vi "Simple Frequency Reader.vi"(8 "error in (no error)":errorcluster) -> (0 "error out":errorcluster)   [LabVIEW 2013]
uses:
  <vilib>/Platform/TimedLoop/XDataNode/wakeup.ctl
  <vilib>/Platform/TimedLoop/XDataNode/XDNodeRunTimeDep.lvlib
  <vilib>/Platform/TimedLoop/XDataNode/nitl_modes.ctl
  <vilib>/Platform/TimedLoop/XDataNode/timing_clust.ctl
  <vilib>/platform/TimedLoop/XDataNode/XDataNode.xnode
  PMU Recorder Light/PMU Recorder Light.lvlib
panel:
  out "Waveform Chart":waveform(sgl)[](graph)
  in  "stop":bool
  in  "Refresh Rate":i64(ring)=200 items=["50 Hz"=20, "20 Hz"=50, "10 Hz"=100, "5 Hz"=200, "2 Hz"=500, "1 Hz"=1000, "Every 2 sec"=2000, "Every 5 sec"=5000, "Every 10 sec"=10000, "Every minute"=60000]
  # "INPUT"
  # "INTERMEDIATE"
  # "OUTPUT"
  # "USAGE:  Start the PRL, configure the input PDC address (IP/Port/PDC ID), press startup and wait until it is connected. \nThen start this VI."
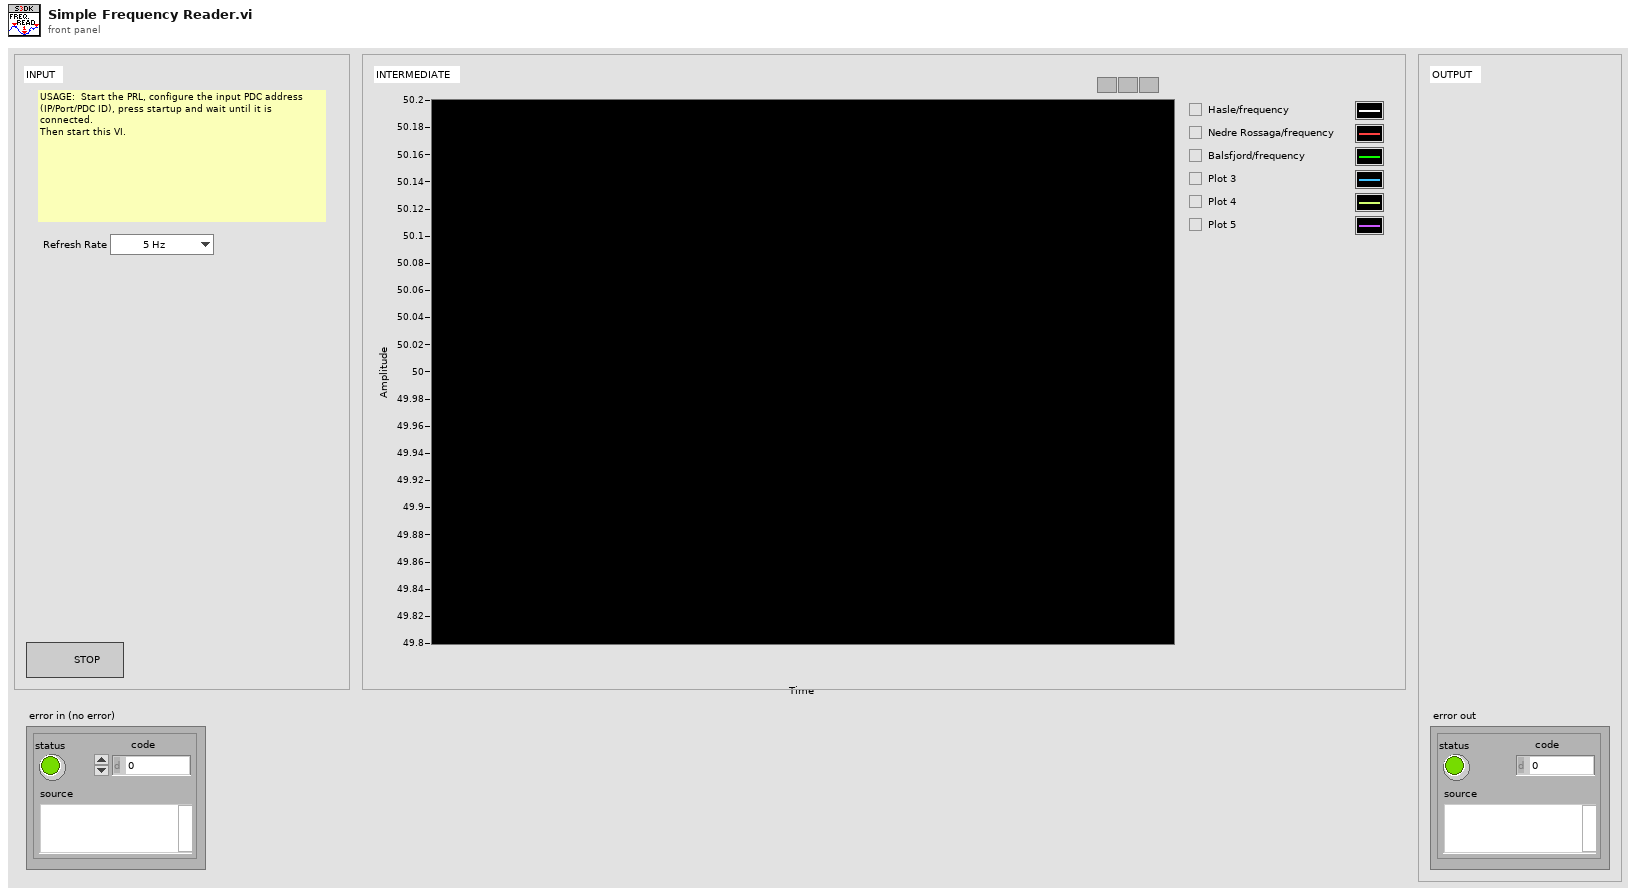
[diagram p1: front panel]
types:
  T1 = enum16{"Filter Signals", "Get All Signal Names", "Select Signals on Name", "Select Frequency Only", "Get Selected Signal Names"}
  T2 = typedef "XDNodeRunTimeDep.lvlib/timing_clust.ctl" = cluster{"Expected End [f-1]":u64, "Actual End [f-1]":u64, "Finished Late? [f-1]":bool, "Expected End [i-1]":u64, "Actual End [i-1]":u64, "Finished Late? [i-1]":bool, "Expected Start [i]":u64, "Actual Start [i]":u64, "Expected Start [f]":u64, "Actual Start [f]":u64, "Source Name":string, "Structure Name":string, "Period":i64, "Deadline":i64, "Offset":i64, "Start":i64, "Priority":i32, "Timeout":i32, "Mode":T3, "Wakeup Reason":T4, "Error":errorcluster, "Source Type":string, "Secondary Source Type":string, "Global End Time":u64, "Global Start Time":u64, "Frame Duration":u64, "Iteration Duration":u64, "Assigned CPU":i32, "I/O Scan Engine Mode":u32}
  T3 = typedef "XDNodeRunTimeDep.lvlib/nitl_modes.ctl" = enum32{"No Change", "Process missed periods, maintain original phase", "Discard missed periods, maintain original phase", "Process missed periods, ignore original phase", "Discard missed periods, ignore original phase"}
  T4 = typedef "XDNodeRunTimeDep.lvlib/wakeup.ctl" = enum32{"Normal", "Aborted", "Asynchronous wakeup", "Timing source error", "Timed loop error", "Timeout"}
  T5 = cluster{"Phasor":string[], "Analog":string[], "Digital":string[]}
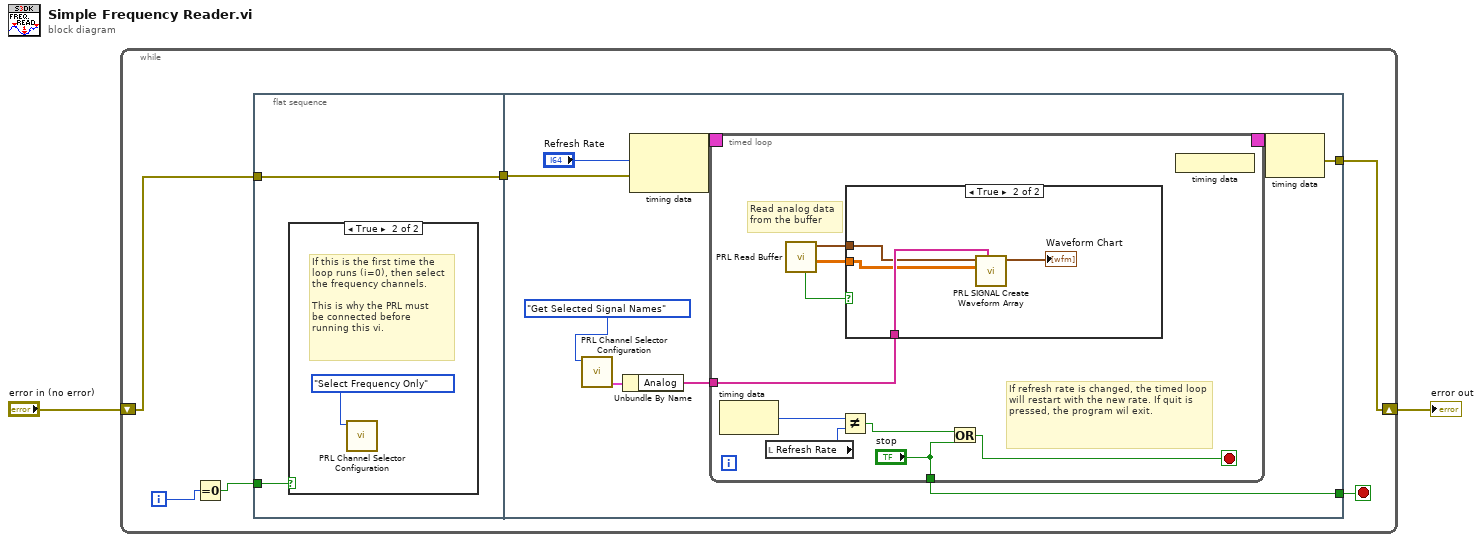
[diagram p0: block diagram]
diagram:
  n1 = while {
    shift-right: [w5] -> w1
    shift-left: "error in (no error)" -> [w3]
    i -> [w7]
    stop <- w8 stop-if-true
    n2 = Equal To 0?(x=w7) -> (x = 0?=w6:bool)
    n3 = flat-sequence {
      tunnel: w6 -> [w10]
      tunnel: [w9] -> w4
      tunnel: w3 -> [w9]
      tunnel: [w17] -> w8
      tunnel: [w13] -> w5
      tunnel: w4 -> [w12]
      frame #0 {
        n4 = case shown="True" w10 {
          frame False {
          }
          frame True {
            # "If this is the first time the\nloop runs (i=0), then select\nthe frequency channels.\n\nThis is why the PRL must\nbe connected before\nrunning this vi."
            n5 = call "PRL Channel Selector Configuration.vi"("Action"=T1."Select Frequency Only") -> ()  [unwired: 10 in, 1 out]
          }
        }
      }
      frame #1 {
        n6 = call "PRL Channel Selector Configuration.vi"("Action"=T1."Get Selected Signal Names") -> ("Signal Names Out"=w15:T5)  [unwired: 10 in]
        n7 = Unbundle By Name(w15) -> ("Analog"=w14:string[])
        n8 = node-c288("Refresh Rate", w12) -> (w20:T2)
        n9 = timed-loop {
          timing: w20 -> [_]
          timing-out: [_] -> w19
          tunnel: ["stop"] -> w17
          tunnel: w14 -> [w21]
          stop <- w27 stop-if-true
          # "Read analog data\nfrom the buffer"
          # "If refresh rate is changed, the timed loop will restart with the new rate. If quit is pressed, the program wil exit."
          n10 = node-c288() -> (w29:i64)  [unwired: 1 in]
          n11 = local read "Refresh Rate"() -> (w28:i64)
          n12 = call "PRL Read Buffer .vi"() -> ("Analog Signals"=w22:sgl[][], "Timestamp"=w23:timestamp[], "Has Data"=w24:bool)  [unwired: 6 in, 3 out]
          n13 = Not Equal?(x=w29, y=w28) -> (x != y?=w26:bool)
          n14 = case shown="True" w24 {
            tunnel: w23 -> [_ w32]
            tunnel: w22 -> [_ w31]
            tunnel: w21 -> [_ w33]
            frame False {
              # "If there is no new data there is no point in sending them to the plot."
            }
            frame True {
              n15 = call "PRL SIGNAL Create Waveform Array.vi"("Signal Names"=w33, "Analog Signals"=w31, "Timestamp"=w32) -> ("Waveform Array"=→"Waveform Chart":waveform(sgl)[])  [unwired: 8 in]
            }
          }
          n16 = Or(x=w26, y="stop") -> (x .or. y?=w27:bool)
          n17 = node-c288() -> ()  [unwired: 1 out]
        }
        n18 = node-c288(w19) -> (w13:errorcluster)
      }
    }
  }
  "error out" <- w1
